vi "Write element.vi"(9 "seconds since 1Jan1904":timestamp, 10 "Variant":variant, 11 "request in":T1 {"node status" items=["Good"=0, "Uncertain"=1073741824, "Uncertain_InitialValue"=1083310080, "Uncertain_LastUsableValue"=1083179008, "Uncertain_SensorNotAccurate"=1083375616, "Uncertain_EngineeringUnitsExceeded"=1083441152, "Bad"=2147483648, "Bad_NoCommunication"=2150694912, "Bad_NotReadable"=2151284736, "Bad_NotWritable"=2151350272, "Bad_OutOfRange"=2151415808, "Bad_WaitingForInitialData"=2150760448]}) -> (3 "request out":T1 {"node status" items=["Good"=0, "Uncertain"=1073741824, "Uncertain_InitialValue"=1083310080, "Uncertain_LastUsableValue"=1083179008, "Uncertain_SensorNotAccurate"=1083375616, "Uncertain_EngineeringUnitsExceeded"=1083441152, "Bad"=2147483648, "Bad_NoCommunication"=2150694912, "Bad_NotReadable"=2151284736, "Bad_NotWritable"=2151350272, "Bad_OutOfRange"=2151415808, "Bad_WaitingForInitialData"=2150760448]})   [LabVIEW 2019, in "OPC addons.lvlib"]
uses:
  <vilib>/OPCUA/controls/Write Variant Request.ctl
  <vilib>/OPCUA/controls/NodeId.ctl
  <vilib>/OPCUA/controls/Write Status.ctl
  OPC addons.lvlib
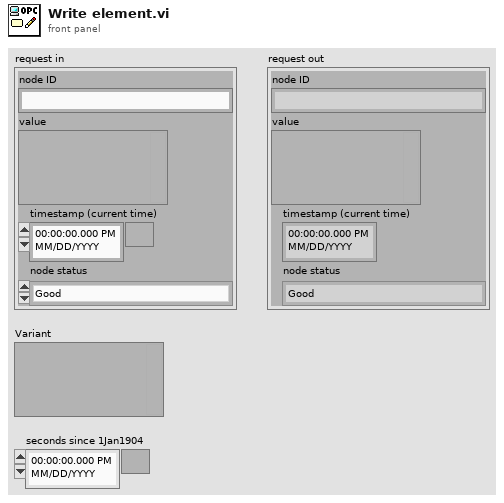
[diagram p1: front panel]
types:
  T1 = typedef "Write Variant Request.ctl" = cluster{"node ID":T2, "value":variant, "timestamp (current time)":timestamp, "node status":T3}
  T2 = typedef "NodeId.ctl" = string
  T3 = typedef "Write Status.ctl" = u32
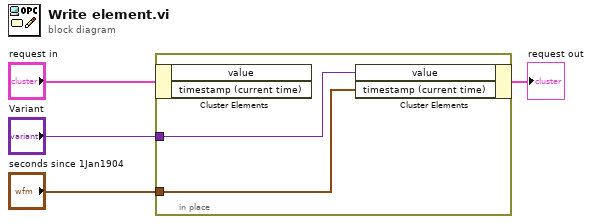
[diagram p0: block diagram]
diagram:
  n1 = in-place {
    in-place-border: "Variant" -> [w6]
    in-place-border: "seconds since 1Jan1904" -> [w5]
    n2 = in-place-cluster #1("request in") -> ()  [unwired: 2 out]
    n3 = in-place-cluster #1("value"=w6, "timestamp (current time)"=w5) -> (→"request out":T1)
  }
